vi "Get Initial LS Data.vi"(8 "Error In":errorcluster, 11 "Path":path) -> (0 "Error Out":errorcluster, 3 "Initial LS Data":T1 {"Opens" format="%#.0f"; "Anomalies (Last Cycle)" format="%#.0f"; "Anomalies/Cycle" format="%#.0f"; "Cycles" format="%#.0f"; "Anomalies Total" format="%#.0f"; "Steps" format="%#.0f"; "Total Cycles" format="%#.0f"})   [LabVIEW 2018]
uses:
  Type Defs/LS Data.ctl
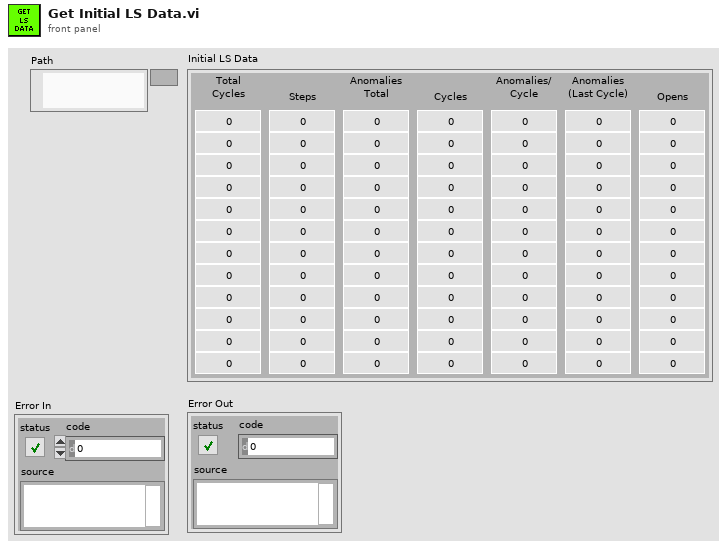
[diagram p1: front panel]
types:
  T1 = typedef "LS Data.ctl" = cluster{"Total Cycles":u32[], "Steps":u32[], "Anomalies Total":i32[], "Cycles":u32[], "Anomalies/Cycle":i32[], "Anomalies (Last Cycle)":i32[], "Opens":i32[]}
  T2 = enum16{"open", "replace", "create", "open or create", "replace or create", "replace or create with confirmation"}
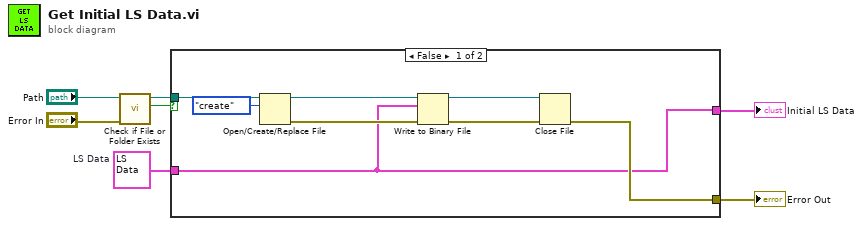
[diagram p0: block diagram]
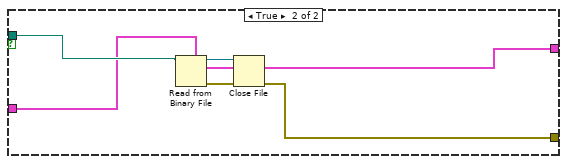
[diagram p2: hidden frame]
diagram:
  w2 = T1 {"Total Cycles"=[0, 0, 0, 0, 0, 0, 0, 0, 0, 0, 0, 0], "Steps"=[0, 0, 0, 0, 0, 0, 0, 0, 0, 0, 0, 0], "Anomalies Total"=[0, 0, 0, 0, 0, 0, 0, 0, 0, 0, 0, 0], "Cycles"=[0, 0, 0, 0, 0, 0, 0, 0, 0, 0, 0, 0], "Anomalies/Cycle"=[0, 0, 0, 0, 0, 0, 0, 0, 0, 0, 0, 0], "Anomalies (Last Cycle)"=[0, 0, 0, 0, 0, 0, 0, 0, 0, 0, 0, 0], "Opens"=[0, 0, 0, 0, 0, 0, 0, 0, 0, 0, 0, 0]}  # LS Data
  n1 = call <vilib>:"Check if File or Folder Exists.vi"("error in (no error)"="Error In", "path"="Path") -> ("file or folder exists?"=w3:bool, "dup path"=w5:path)  [unwired: 7 in, 1 out]
  n2 = case shown="False" w3 {
    tunnel: w5 -> [w15 w21]
    tunnel: [w8 w20] -> w1
    tunnel: [w12 w19] -> w4
    tunnel: w2 -> [w8 w16]
    frame False {
      n3 = Open/Create/Replace File(file path (use dialog)=w15, operation (0:open)=T2."create") -> (refnum out=w10:refnum<file>, error out=w9:errorcluster)  [unwired: 4 in, 1 out]
      n4 = Write to Binary File(file (use dialog)=w10, data=w8, error in=w9) -> (refnum out=w13:refnum<file>, error out=w14:errorcluster)  [unwired: 3 in, 1 out]
      n5 = Close File(refnum=w13, error in=w14) -> (error out=w12:errorcluster)  [unwired: 1 out]
    }
    frame True {
      n6 = Read from Binary File(5:w16, 11:w21) -> (0:w17:errorcluster, 2:w20:T1, 3:w18:refnum<file>)  [unwired: 4 in, 1 out]
      n7 = Close File(refnum=w18, error in=w17) -> (error out=w19:errorcluster)  [unwired: 1 out]
    }
  }
  "Error Out" <- w4
  "Initial LS Data" <- w1
